vi "偏置计算.vi"(7 "实时测量数据":string[][](array[string])=[["时间", "温度（℃）", "压力（KPa）", "电压1（V）", "桥压1（V）", "电压2（V）", "桥压2（V）", "电压3（V）", "桥压3（V）", "电压4（V）", "桥压4（V）", "电压5（V）", "桥压5（V）"], ["", "", "1", " ", "2", " ", "3", " ", "4", " ", "", "", ""], ["", "", "正行程", "", "", "", "", "", "", "", "", "", ""], ["17:06:40", "11.900000", "199.921", "-6.32\n-6.32\n", "7.8325\n", "5\n67000E-6", "-2.844000E-6", "6", "-3.109000E-6", "7", "-2.897000E-6", "8", ""], ["17:07:13", "12.000000", "299.9351", "51.474", "7.8338", "-3.013000E-6", "-3.491000E-6", "-2.918000E-6", "-3.332000E-6", "-2.780000E-6", "-3.204000E-6", "", ""], ["17:07:36", "12.000000", "399.96", "110.353", "7.8346", "-3.120000E-6", "-3.289000E-6", "-2.960000E-6", "-3.141000E-6", "-3.385000E-6", "-2.844000E-6", "", ""], ["", "", "反行程", "", "", "", "", "", "", "", "", "", ""], ["17:08:20", "12.000000", "400.0285", "110.353", "7.8346", "-3.120000E-6", "-3.342000E-6", "-3.162000E-6", "-3.194000E-6", "-3.056000E-6", "-3.194000E-6", "", ""], ["17:08:45", "12.000000", "300.0653", "52.283", "7.8332", "-3.342000E-6", "-3.321000E-6", "-3.013000E-6", "-3.311000E-6", "-3.300000E-6", "-3.162000E-6", "", ""], ["17:09:22", "12.000000", "200.0595", "-6.299", "7.8346", "-2.907000E-6", "-3.194000E-6", "-3.257000E-6", "-3.204000E-6", "-3.077000E-6", "-2.971000E-6", "", ""], ["", "", "正行程", "", "", "", "", "", "", "", "", "", ""], ["17:13:30", "12.100000", "199.9466", "-7.532", "8.8568", "-3.671000E-6", "-3.353000E-6", "-3.799000E-6", "-3.565000E-6", "-3.746000E-6", "-3.374000E-6", "", ""], ["17:13:53", "12.100000", "299.95", "53.539", "8.8574", "-3.311000E-6", "-3.502000E-6", "-3.364000E-6", "-3.618000E-6", "-3.120000E-6", "-3.406000E-6", "", ""], ["17:14:26", "12.100000", "399.8962", "116.27", "8.8567", "-3.756000E-6", "-3.830000E-6", "-3.427000E-6", "-3.597000E-6", "-3.777000E-6", "-3.576000E-6", "", ""], ["", "", "反行程", "", "", "", "", "", "", "", "", "", ""], ["17:15:01", "12.100000", "399.9835", "116.27", "8.8567", "-3.395000E-6", "-3.289000E-6", "-3.120000E-6", "-3.502000E-6", "-3.427000E-6", "-3.353000E-6", "", ""], ["17:15:38", "12.100000", "299.9459", "54.318", "8.8552", "-3.512000E-6", "-3.650000E-6", "-3.809000E-6", "-3.480000E-6", "-3.300000E-6", "-3.767000E-6", "", ""], ["17:16:15", "12.100000", "199.9841", "-7.516", "8.8564", "-3.629000E-6", "-3.608000E-6", "-3.767000E-6", "-3.639000E-6", "-3.417000E-6", "-3.406000E-6", "", ""], ["-3.0\n67000E-6", "-3.0\n67000E-6", "0\n67000E-6", "-3.0\n67000E-6", "-3.0\n67000E-6", "-3.0\n67000E-6", "-3.0\n67000E-6", "-3.0\n67000E-6", "-3.0\n67000E-6", "-3.0\n67000E-6", "-3.0\n67000E-6", "-3.0\n67000E-6", "-3.0\n67000E-6"], ["-3.0\n67000E-6", "-3.0\n67000E-6", "1\n67000E-6", "-3.0\n67000E-6", "-3.0\n67000E-6", "-3.0\n67000E-6", "-3.0\n67000E-6", "-3.0\n67000E-6", "-3.0\n67000E-6", "-3.0\n67000E-6", "-3.0\n67000E-6", "-3.0\n67000E-6", "-3.0\n67000E-6"], ["-3.0\n67000E-6", "-3.0\n67000E-6", "2\n67000E-6", "-3.0\n67000E-6", "-3.0\n67000E-6", "-3.0\n67000E-6", "-3.0\n67000E-6", "-3.0\n67000E-6", "-3.0\n67000E-6", "-3.0\n67000E-6", "-3.0\n67000E-6", "-3.0\n67000E-6", "-3.0\n67000E-6"], ["-3.0\n67000E-6", "-3.0\n67000E-6", "3\n67000E-6", "-3.0\n67000E-6", "-3.0\n67000E-6", "-3.0\n67000E-6", "-3.0\n67000E-6", "-3.0\n67000E-6", "-3.0\n67000E-6", "-3.0\n67000E-6", "-3.0\n67000E-6", "-3.0\n67000E-6", "-3.0\n67000E-6"], ["-3.0\n67000E-6", "-3.0\n67000E-6", "0\n67000E-6", "-3.0\n67000E-6", "-3.0\n67000E-6", "-3.0\n67000E-6", "-3.0\n67000E-6", "-3.0\n67000E-6", "-3.0\n67000E-6", "-3.0\n67000E-6", "-3.0\n67000E-6", "-3.0\n67000E-6", "-3.0\n67000E-6"], ["-3.0\n67000E-6", "-3.0\n67000E-6", "3\n67000E-6", "-3.0\n67000E-6", "-3.0\n67000E-6", "-3.0\n67000E-6", "-3.0\n67000E-6", "-3.0\n67000E-6", "-3.0\n67000E-6", "-3.0\n67000E-6", "-3.0\n67000E-6", "-3.0\n67000E-6", "-3.0\n67000E-6"], ["-3.0\n67000E-6", "-3.0\n67000E-6", "2\n67000E-6", "-3.0\n67000E-6", "-3.0\n67000E-6", "-3.0\n67000E-6", "-3.0\n67000E-6", "-3.0\n67000E-6", "-3.0\n67000E-6", "-3.0\n67000E-6", "-3.0\n67000E-6", "-3.0\n67000E-6", "-3.0\n67000E-6"], ["-3.0\n67000E-6", "-3.0\n67000E-6", "1\n67000E-6", "-3.0\n67000E-6", "-3.0\n67000E-6", "-3.0\n67000E-6", "-3.0\n67000E-6", "-3.0\n67000E-6", "-3.0\n67000E-6", "-3.0\n67000E-6", "-3.0\n67000E-6", "-3.0\n67000E-6", "-3.0\n67000E-6"]], 8 "压力点个数":dbl=6.0, 10 "理论K":dbl=306.667, 11 "R5-1":dbl) -> (1 "拟合":string[](array[string]), 3 "RX":dbl[](array[numeric]))   [LabVIEW 2017]
uses:
  044b461c-7e22-40d5-9c00-1427d5951afe.vi
  8a9c416f-a0c3-482a-b640-094a18977def.vi
  46fd01af-a86e-4f15-bd5a-be8893c0a065.vi
  <vilib>/Array/Sort 2D Array - Pop Stack.vi
  <vilib>/Array/Sort 2D Array - Push Stack.vi
  <vilib>/Analysis/NI_AALPro.lvlib
panel:
  out "拟合 5":string
  out "拟合 4":string
  out "拟合 3":string
  out "拟合 2":string
  out "拟合1":string
  out "intercept 5":dbl caption="截距"
  out "slope 5":dbl caption="斜率"
  out "intercept 4":dbl caption="截距"
  out "slope 4":dbl caption="斜率"
  out "intercept 3":dbl caption="截距"
  out "slope 3":dbl caption="斜率"
  out "intercept 2":dbl caption="截距"
  out "slope 2":dbl caption="斜率"
  out "intercept":dbl caption="截距"
  out "slope":dbl caption="斜率"
  out "5":dbl[](array[numeric])
  out "4":dbl[](array[numeric])
  out "3":dbl[](array[numeric])
  out "2":dbl[](array[numeric])
  out "1":dbl[](array[numeric])
  out "压力":dbl[](array[numeric])
  out "平均":dbl[][](array[numeric])
  out "已删除元素的数组子集":string[][](array[string])
  in  "数据":dbl[][](array[numeric])=[[199.921, 4.0, 7.8325, 4.0, -2.844e-06, -3.3e-06, -3.109e-06, -3.045e-06, -2.897e-06, 1.0, 0.0], [299.9351, 4.0, 7.8338, 1.0, -3.491e-06, -2.918e-06, -3.332e-06, -2.78e-06, -3.204e-06, 0.0, 0.0], [399.96, 4.0, 7.8346, -3.12e-06, -3.289e-06, -2.96e-06, -3.141e-06, -3.385e-06, -2.844e-06, 0.0, 0.0], [400.0285, -4.0, 7.8346, 0.0, -3.342e-06, -3.162e-06, -3.194e-06, -3.056e-06, -3.194e-06, 0.0, 0.0], [300.0653, -4.0, 7.8332, -3.342e-06, -3.321e-06, -3.013e-06, -3.311e-06, -3.3e-06, -3.162e-06, 0.0, 0.0], [200.0595, -4.0, 7.8346, -2.907e-06, -3.194e-06, -3.257e-06, -3.204e-06, -3.077e-06, -2.971e-06, 0.0, 0.0], [199.9466, 4.0, 8.8568, 5.0, -3.353e-06, -3.799e-06, -3.565e-06, -3.746e-06, -3.374e-06, 0.0, 0.0], [299.95, 4.0, 8.8574, -3.311e-06, -3.502e-06, -3.364e-06, -3.618e-06, -3.12e-06, -3.406e-06, 0.0, 0.0], [399.8962, 4.0, 8.8567, -3.756e-06, -3.83e-06, -3.427e-06, -3.597e-06, -3.777e-06, -3.576e-06, 0.0, 0.0], [399.9835, -4.0, 8.8567, 0.0, -3.289e-06, -3.12e-06, -3.502e-06, -3.427e-06, -3.353e-06, 0.0, 0.0], [299.9459, -4.0, 8.8552, -3.512e-06, -3.65e-06, -3.809e-06, -3.48e-06, -3.3e-06, -3.767e-06, 0.0, 0.0], [199.9841, -4.0, 8.8564, -3.629e-06, -3.608e-06, -3.767e-06, -3.639e-06, -3.417e-06, -3.406e-06, 0.0, 0.0], [200.0, 4.0, 0.0, 1.0, 0.0, 0.0, 0.0, 0.0, 0.0, 0.0, 0.0], [300.0, 4.0, 0.0, 2.0, 0.0, 0.0, 0.0, 0.0, 0.0, 0.0, 0.0], [400.0, 4.0, 0.0, 3.0, 0.0, 0.0, 0.0, 0.0, 0.0, 0.0, 0.0], [400.0, -4.0, 0.0, 20.0, 0.0, 0.0, 0.0, 0.0, 0.0, 0.0, 0.0], [300.0, -4.0, 0.0, 5.0, 0.0, 0.0, 0.0, 0.0, 0.0, 0.0, 0.0], [200.0, -4.0, 0.0, 6.0, 0.0, 0.0, 0.0, 0.0, 0.0, 0.0, 0.0], [200.0, 0.0, 0.0, 7.0, 0.0, 0.0, 0.0, 0.0, 0.0, 0.0, 0.0], [300.0, 0.0, 0.0, 8.0, 0.0, 0.0, 0.0, 0.0, 0.0, 0.0, 0.0], [400.0, 0.0, 0.0, 9.0, 0.0, 0.0, 0.0, 0.0, 0.0, 0.0, 0.0], [400.0, -7.0, 0.0, 10.0, 0.0, 0.0, 0.0, 0.0, 0.0, 0.0, 0.0], [300.0, -7.0, 0.0, 11.0, 0.0, 0.0, 0.0, 0.0, 0.0, 0.0, 0.0], [200.0, -7.0, 0.0, 12.0, 0.0, 0.0, 0.0, 0.0, 0.0, 0.0, 0.0], [0.0, 0.0, 0.0, 13.0, 0.0, 0.0, 0.0, 0.0, 0.0, 0.0, 0.0], [0.0, 0.0, 0.0, 14.0, 0.0, 0.0, 0.0, 0.0, 0.0, 0.0, 0.0], [0.0, 0.0, 0.0, 15.0, 0.0, 0.0, 0.0, 0.0, 0.0, 0.0, 0.0], [0.0, -7.0, 0.0, 16.0, 0.0, 0.0, 0.0, 0.0, 0.0, 0.0, 0.0], [0.0, -7.0, 0.0, 17.0, 0.0, 0.0, 0.0, 0.0, 0.0, 0.0, 0.0], [0.0, -7.0, 0.0, 18.0, 0.0, 0.0, 0.0, 0.0, 0.0, 0.0, 0.0], [0.0, 0.0, 0.0, 19.0, 0.0, 0.0, 0.0, 0.0, 0.0, 0.0, 0.0], [0.0, 0.0, 0.0, 20.0, 0.0, 0.0, 0.0, 0.0, 0.0, 0.0, 0.0], [0.0, 0.0, 0.0, 21.0, 0.0, 0.0, 0.0, 0.0, 0.0, 0.0, 0.0], [0.0, -7.0, 0.0, 22.0, 0.0, 0.0, 0.0, 0.0, 0.0, 0.0, 0.0], [0.0, -7.0, 0.0, 23.0, 0.0, 0.0, 0.0, 0.0, 0.0, 0.0, 0.0], [0.0, -7.0, 0.0, 24.0, 0.0, 0.0, 0.0, 0.0, 0.0, 0.0, 0.0], [0.0, 0.0, 0.0, 25.0, 0.0, 0.0, 0.0, 0.0, 0.0, 0.0, 0.0], [0.0, 0.0, 0.0, 26.0, 0.0, 0.0, 0.0, 0.0, 0.0, 0.0, 0.0], [0.0, 0.0, 0.0, 27.0, 0.0, 0.0, 0.0, 0.0, 0.0, 0.0, 0.0]]
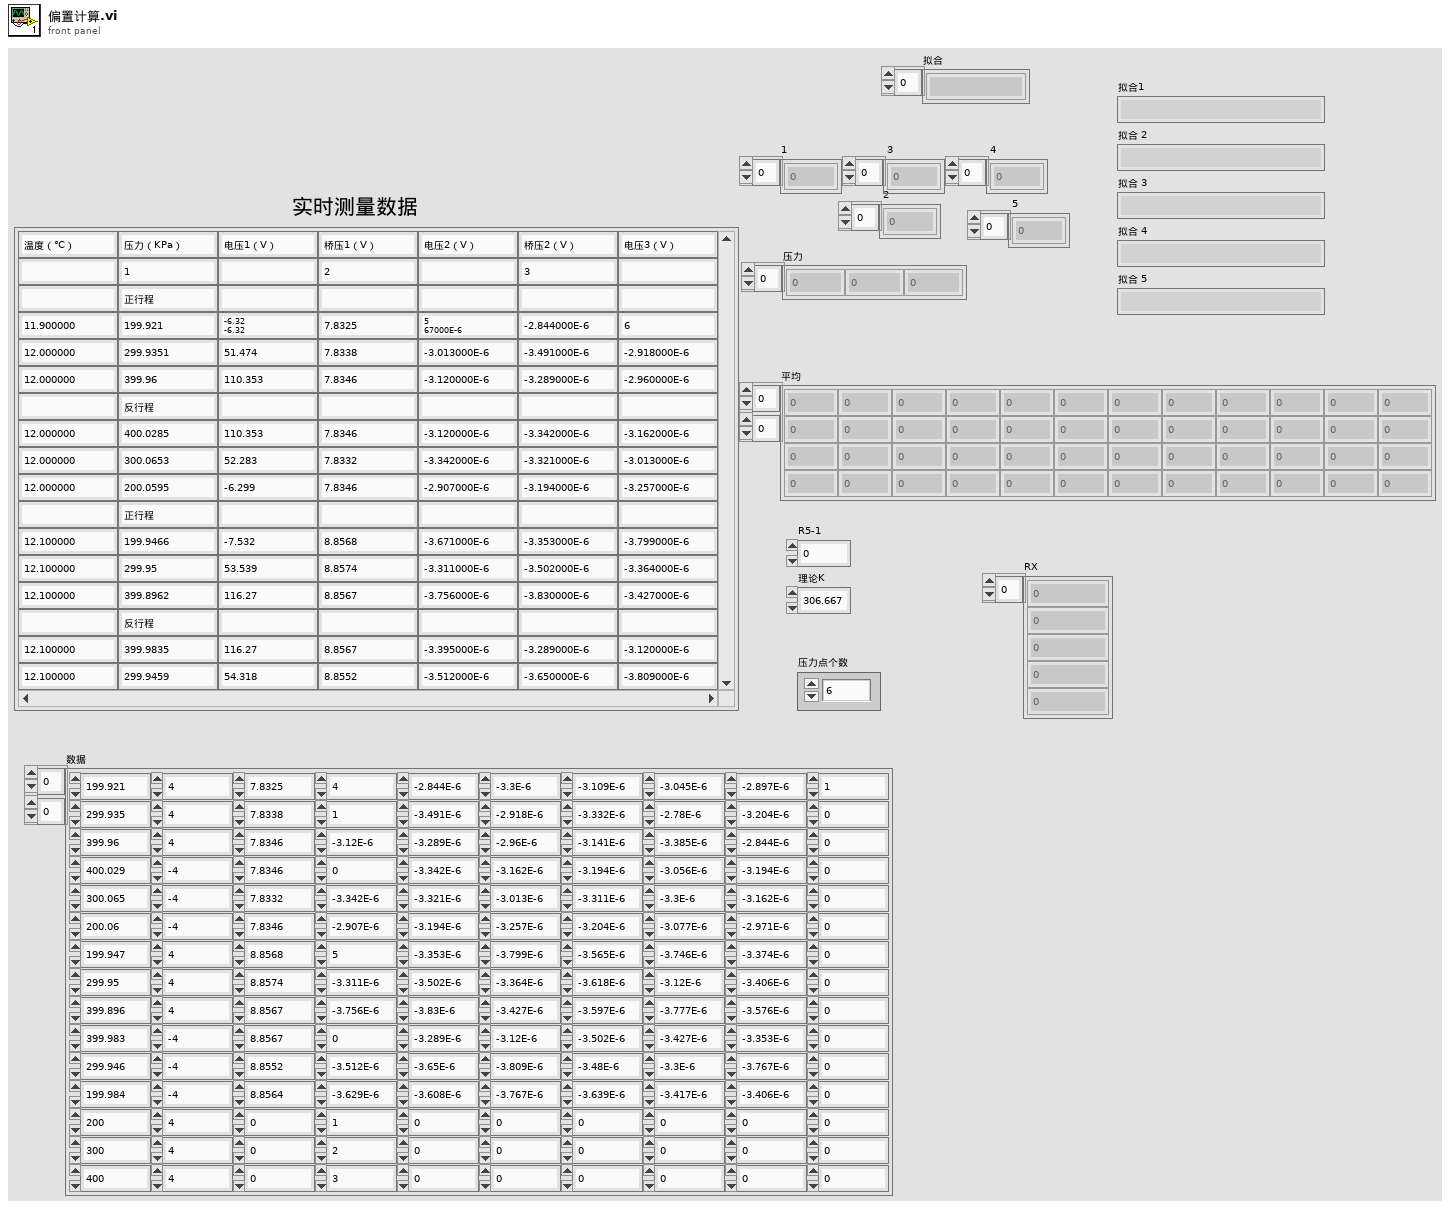
[diagram p1: front panel]
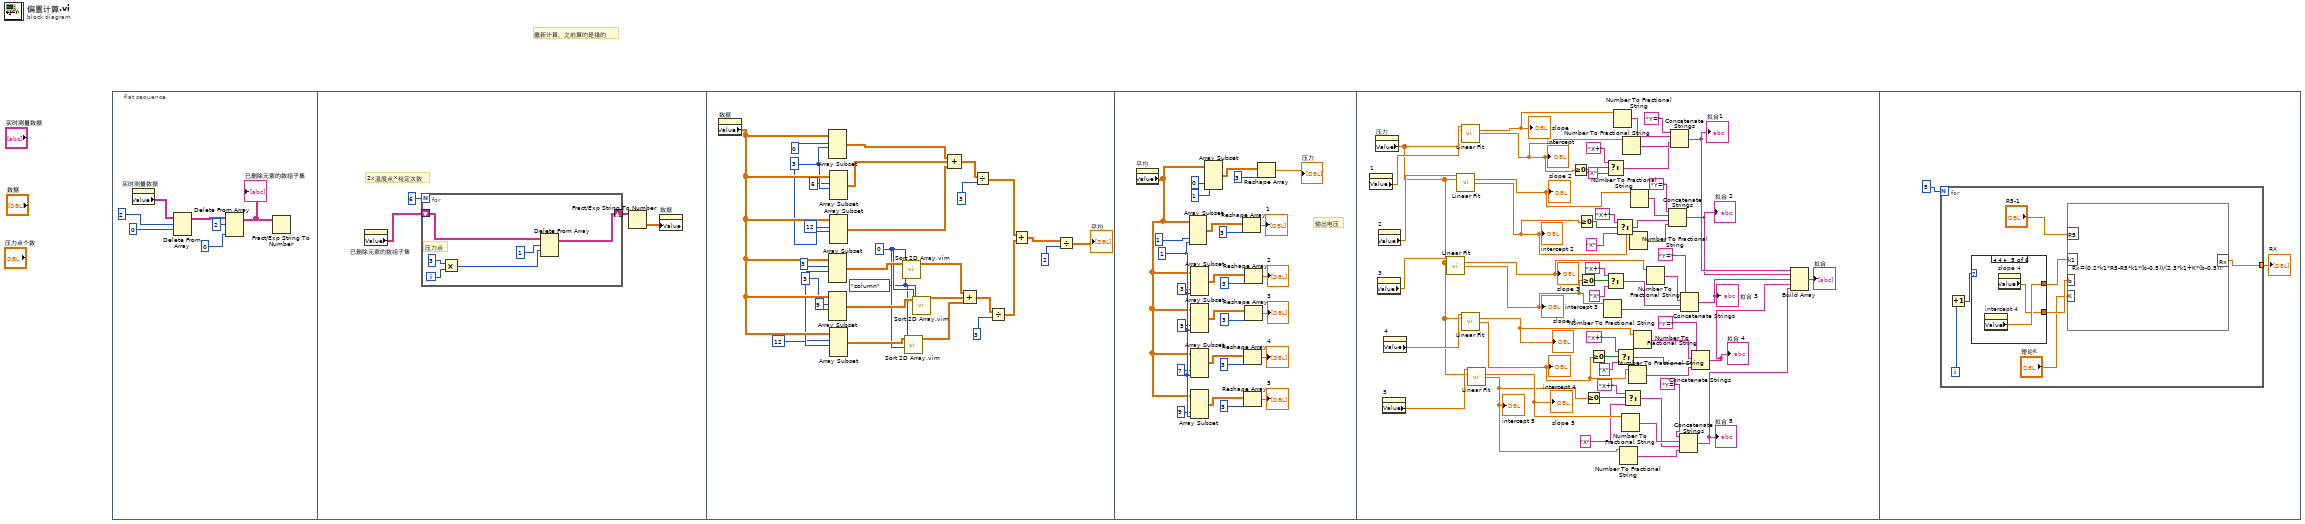
[diagram p0: block diagram]
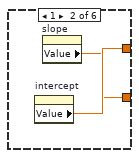
[diagram p3: hidden frame]
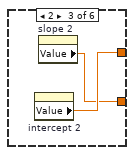
[diagram p4: hidden frame]
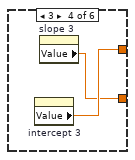
[diagram p5: hidden frame]
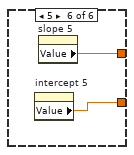
[diagram p6: hidden frame]
diagram:
  # "重新计算、之前算的是错的"
  n1 = flat-sequence {
    frame #0 {
      n2 = property on="实时测量数据" class="Arr (严格)"() -> ("Value"=w5:string[][])  [unwired: 2 in, 2 out]
      n3 = Delete From Array(array=w5, length=2 ("长度"), index (row)=0 ("索引 (行)")) -> (array with subset deleted=w6:string[][])  [unwired: 1 in, 1 out]
      n4 = Delete From Array(array=w6, length=2 ("长度"), index (col)=0 ("禁用的索引 (列)")) -> (array with subset deleted=w7:string[][])  [unwired: 1 in, 1 out]
      "已删除元素的数组子集" <- w7
      n5 = Fract/Exp String To Number(string=w7) -> ()  [unwired: 3 in, 2 out]
    }
    frame #1 {
      # "2x温度点×检定次数"
      n6 = property on="已删除元素的数组子集" class="Arr (严格)"() -> ("Value"=w9:string[][])  [unwired: 2 in, 2 out]
      n7 = for {
        N: 6 -> [_]
        shift-right: [w13] -> w10
        shift-left: w9 -> [w12]
        i -> [w16]
        # "压力点"
        n8 = Multiply(x=3, y=w16) -> (x*y=w15:i32)
        n9 = Delete From Array(array=w12, length=1 ("长度"), index (row)=w15) -> (array with subset deleted=w13:string[][])  [unwired: 1 in, 1 out]
      }
      n10 = Fract/Exp String To Number(string=w10) -> (number=w11:dbl[][])  [unwired: 3 in, 1 out]
      n11 = property on="数据" class="Arr (严格)"("Value"=w11) -> ()  [unwired: 2 in, 2 out]
    }
    frame #2 {
      w27 = 0 ("index")
      w26 = enum16{"column", "row"}."column" ("dimension to index (column)")
      w24 = 3
      w20 = 3 ("长度")
      n12 = property on="数据" class="Arr (严格)"() -> ("Value"=w31:dbl[][])  [unwired: 2 in, 2 out]
      n13 = Array Subset(array=w31, index (row)=9 ("索引"), length (row)=w24) -> (w33:dbl[][])  [unwired: 2 in]
      n14 = Array Subset(array=w31, index (row)=0 ("索引"), length (row)=w20) -> (w35:dbl[][])  [unwired: 2 in]
      n15 = Array Subset(array=w31, index (row)=3 ("索引"), length (row)=w24) -> (w32:dbl[][])  [unwired: 2 in]
      n16 = Array Subset(array=w31, index (row)=6 ("索引"), length (row)=w20) -> (w36:dbl[][])  [unwired: 2 in]
      n17 = Array Subset(array=w31, index (row)=12 ("索引"), length (row)=w20) -> (w37:dbl[][])  [unwired: 2 in]
      n18 = Array Subset(array=w31, index (row)=12 ("索引"), length (row)=w24) -> (w34:dbl[][])  [unwired: 2 in]
      n19 = call "Sort 2D Array.vim"("index"=w27, "dimension to index (column)"=w26, "2D array"=w32) -> ("sorted 2D array"=w40:dbl[][])  [unwired: 7 in, 1 out]
      n20 = call "Sort 2D Array.vim"("index"=w27, "dimension to index (column)"=w26, "2D array"=w34) -> ("sorted 2D array"=w42:dbl[][])  [unwired: 7 in, 1 out]
      n21 = call "Sort 2D Array.vim"("index"=w27, "dimension to index (column)"=w26, "2D array"=w33) -> ("sorted 2D array"=w41:dbl[][])  [unwired: 7 in, 1 out]
      n22 = Compound Arithmetic op=ADD(w35, w36, w37) -> (w38:dbl[][])
      n23 = Compound Arithmetic op=ADD(w40, w41, w42) -> (w39:dbl[][])
      n24 = Divide(x=w38, y=3) -> (x/y=w43:dbl[][])
      n25 = Divide(x=w39, y=3) -> (x/y=w44:dbl[][])
      n26 = Add(x=w43, y=w44) -> (x+y=w45:dbl[][])
      n27 = Divide(x=w45, y=2) -> (x/y=→"平均":dbl[][])
    }
    frame #3 {
      w57 = 1 ("长度")
      # "输出电压"
      n28 = property on="平均" class="Arr (严格)"() -> ("Value"=w56:dbl[][])  [unwired: 2 in, 2 out]
      n29 = Array Subset(array=w56, index (col)=1 ("索引"), length (col)=w57) -> (w67:dbl[][])  [unwired: 2 in]
      n30 = Array Subset(array=w56, index (col)=7 ("索引"), length (col)=w57) -> (w61:dbl[][])  [unwired: 2 in]
      n31 = Array Subset(array=w56, index (col)=9 ("索引"), length (col)=w57) -> (w59:dbl[][])  [unwired: 2 in]
      n32 = Array Subset(array=w56, index (col)=3 ("索引"), length (col)=w57) -> (w65:dbl[][])  [unwired: 2 in]
      n33 = Array Subset(array=w56, index (col)=5 ("索引"), length (col)=w57) -> (w63:dbl[][])  [unwired: 2 in]
      n34 = Array Subset(array=w56, index (col)=0 ("索引"), length (col)=1 ("长度")) -> (w71:dbl[][])  [unwired: 2 in]
      n35 = Reshape Array(w67, 3 ("维数大小")) -> (→"1":dbl[])
      n36 = Reshape Array(w61, 3 ("维数大小")) -> (→"4":dbl[])
      n37 = Reshape Array(w59, 3 ("维数大小")) -> (→"5":dbl[])
      n38 = Reshape Array(w65, 3 ("维数大小")) -> (→"2":dbl[])
      n39 = Reshape Array(w63, 3 ("维数大小")) -> (→"3":dbl[])
      n40 = Reshape Array(w71, 3 ("维数大小")) -> (→"压力":dbl[])
    }
    frame #4 {
      n41 = property on="1" class="Arr (严格)"() -> ("Value"=w126:dbl[])  [unwired: 2 in, 2 out]
      n42 = property on="压力" class="Arr (严格)"() -> ("Value"=w125:dbl[])  [unwired: 2 in, 2 out]
      n43 = property on="3" class="Arr (严格)"() -> ("Value"=w129:dbl[])  [unwired: 2 in, 2 out]
      n44 = property on="2" class="Arr (严格)"() -> ("Value"=w130:dbl[])  [unwired: 2 in, 2 out]
      n45 = property on="5" class="Arr (严格)"() -> ("Value"=w127:dbl[])  [unwired: 2 in, 2 out]
      n46 = property on="4" class="Arr (严格)"() -> ("Value"=w128:dbl[])  [unwired: 2 in, 2 out]
      n47 = call <vilib>:"Linear Fit.vi"("Y"=w129, "X"=w125) -> ("slope"=w113:dbl, "intercept"=w92:dbl)  [unwired: 9 in, 3 out]
      "slope 3" <- w113
      "intercept 3" <- w92
      n48 = call <vilib>:"Linear Fit.vi"("Y"=w130, "X"=w125) -> ("slope"=w115:dbl, "intercept"=w93:dbl)  [unwired: 9 in, 3 out]
      "slope 2" <- w115
      "intercept 2" <- w93
      n49 = call <vilib>:"Linear Fit.vi"("Y"=w126, "X"=w125) -> ("slope"=w119:dbl, "intercept"=w94:dbl)  [unwired: 9 in, 3 out]
      "slope" <- w119
      "intercept" <- w94
      n50 = call <vilib>:"Linear Fit.vi"("Y"=w128, "X"=w125) -> ("slope"=w110:dbl, "intercept"=w91:dbl)  [unwired: 9 in, 3 out]
      "slope 4" <- w110
      "intercept 4" <- w91
      n51 = call <vilib>:"Linear Fit.vi"("Y"=w127, "X"=w125) -> ("slope"=w107:dbl, "intercept"=w90:dbl)  [unwired: 9 in, 3 out]
      "slope 5" <- w107
      "intercept 5" <- w90
      n52 = Greater Or Equal To 0?(x=w94) -> (x >= 0?=w124:bool)
      n53 = Greater Or Equal To 0?(x=w93) -> (x >= 0?=w123:bool)
      n54 = Greater Or Equal To 0?(x=w92) -> (x >= 0?=w122:bool)
      n55 = Greater Or Equal To 0?(x=w90) -> (x >= 0?=w120:bool)
      n56 = Greater Or Equal To 0?(x=w91) -> (x >= 0?=w121:bool)
      n57 = Number To Fractional String(number=w92) -> (F-format string=w85:string)  [unwired: 3 in]
      n58 = Select(t="X+", s=w124, f="X") -> (s? t:f=w88:string)
      n59 = Select(t="X+", s=w122, f="X") -> (s? t:f=w84:string)
      n60 = Number To Fractional String(number=w119) -> (F-format string=w118:string)  [unwired: 3 in]
      n61 = Select(t="X+", s=w123, f="X") -> (s? t:f=w87:string)
      n62 = Select(t="X+", s=w121, f="X") -> (s? t:f=w82:string)
      n63 = Number To Fractional String(number=w90) -> (F-format string=w80:string)  [unwired: 3 in]
      n64 = Number To Fractional String(number=w107) -> (F-format string=w105:string)  [unwired: 3 in]
      n65 = Number To Fractional String(number=w94) -> (F-format string=w89:string)  [unwired: 3 in]
      n66 = Select(t="X+", s=w120, f="X") -> (s? t:f=w81:string)
      n67 = Number To Fractional String(number=w91) -> (F-format string=w83:string)  [unwired: 3 in]
      n68 = Number To Fractional String(number=w93) -> (F-format string=w86:string)  [unwired: 3 in]
      n69 = Number To Fractional String(number=w115) -> (F-format string=w114:string)  [unwired: 3 in]
      n70 = Number To Fractional String(number=w110) -> (F-format string=w109:string)  [unwired: 3 in]
      n71 = Number To Fractional String(number=w113) -> (F-format string=w111:string)  [unwired: 3 in]
      n72 = Concatenate Strings("Y=", w114, w87, w86) -> (w78:string)
      "拟合 2" <- w78
      n73 = Concatenate Strings("Y=", w118, w88, w89) -> (w79:string)
      "拟合1" <- w79
      n74 = Concatenate Strings("Y=", w105, w81, w80) -> (w75:string)
      "拟合 5" <- w75
      n75 = Concatenate Strings("Y=", w111, w84, w85) -> (w77:string)
      "拟合 3" <- w77
      n76 = Concatenate Strings("Y=", w109, w82, w83) -> (w76:string)
      "拟合 4" <- w76
      n77 = Build Array(w79, w78, w77, w76, w75) -> (→"拟合":string[])
    }
    frame #5 {
      n78 = for {
        N: 5 -> [_]
        tunnel: [w135] -> w131 mode=indexing
        i -> [w138]
        n79 = Increment(x=w138) -> (x+1=w139:i32)
        n80 = case shown="4" w139 {
          tunnel: [_ w140 w142 w144 w146 w149] -> w137
          tunnel: [_ w141 w143 w145 w147 w148] -> w136
          frame 6, Default {
          }
          frame 1 {
            n81 = property on="intercept" class="DigNum (严格)"() -> ("Value"=w141:dbl)  [unwired: 2 in, 2 out]
            n82 = property on="slope" class="DigNum (严格)"() -> ("Value"=w140:dbl)  [unwired: 2 in, 2 out]
          }
          frame 2 {
            n83 = property on="intercept 2" class="DigNum (严格)"() -> ("Value"=w143:dbl)  [unwired: 2 in, 2 out]
            n84 = property on="slope 2" class="DigNum (严格)"() -> ("Value"=w142:dbl)  [unwired: 2 in, 2 out]
          }
          frame 3 {
            n85 = property on="intercept 3" class="DigNum (严格)"() -> ("Value"=w145:dbl)  [unwired: 2 in, 2 out]
            n86 = property on="slope 3" class="DigNum (严格)"() -> ("Value"=w144:dbl)  [unwired: 2 in, 2 out]
          }
          frame 4 {
            n87 = property on="intercept 4" class="DigNum (严格)"() -> ("Value"=w147:dbl)  [unwired: 2 in, 2 out]
            n88 = property on="slope 4" class="DigNum (严格)"() -> ("Value"=w146:dbl)  [unwired: 2 in, 2 out]
          }
          frame 5 {
            n89 = property on="intercept 5" class="DigNum (严格)"() -> ("Value"=w149:dbl)  [unwired: 2 in, 2 out]
            n90 = property on="slope 5" class="DigNum (严格)"() -> ("Value"=w148:dbl)  [unwired: 2 in, 2 out]
          }
        }
        n91 = formula code="Rx=(0.2*k1*R5-R5*k1*(b-0.5))/(2.3*k1+K*(b-0.5));"("k1"=w136, "R5"="R5-1", "K"="理论K", "b"=w137) -> ("Rx"=w135:dbl)
      }
      "RX" <- w131
    }
  }
